vi "PUMP_feedback_P_FR.vi"(4 "Allow email":bool, 5 "FR Data":cluster{"time (s)":dbl, "volume (µl)":dbl}, 6 "t0":dbl, 7 "FRP":T1, 8 "error in":errorcluster, 9 "MFCS_EZ":T2, 10 "Volume setpoint":dbl, 11 "FR setpoint":dbl) -> (0 "error out":errorcluster, 1 "Allow email out":bool, 2 "FR Data OUT":cluster{"time (s)":dbl, "volume (µl)":dbl}, 3 "volume reached?":bool)   [LabVIEW 2015]
uses:
  <userlib>/Fluigent/Fluigent MFCS/FluigentMFCS_Full.llb/_EZmfcsRefNum.ctl
  <userlib>/Fluigent/Fluigent MFCS/FluigentMFCS_Full.llb/_EZmfcsEnum.ctl
  <userlib>/Fluigent/Fluigent FRP/FluigentFRP.llb/_frpEnum.ctl
  <userlib>/Fluigent/Fluigent MFCS/FluigentMFCS_Full.llb/MFCS_EZ Write Channel Pressure.vi
  GLOBAL/Global_MAIN.vi
panel:
  out "error out MAIL":errorcluster
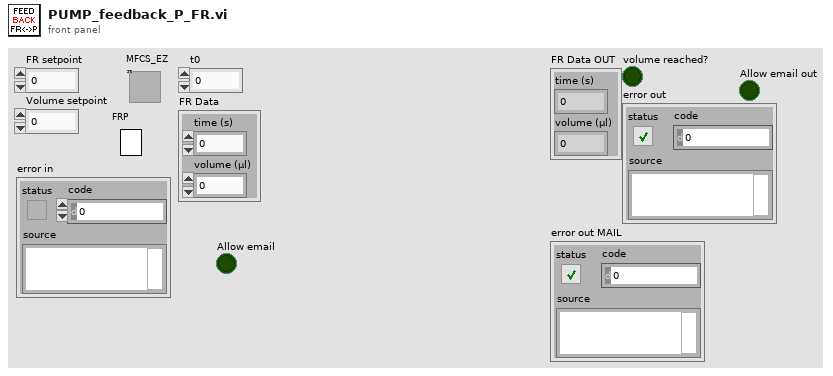
[diagram p1: front panel]
types:
  T1 = typedef "_frpRefNum" = refnum<k1>
  T2 = typedef "_EZmfcsRefNum.ctl" = refnum<k1>
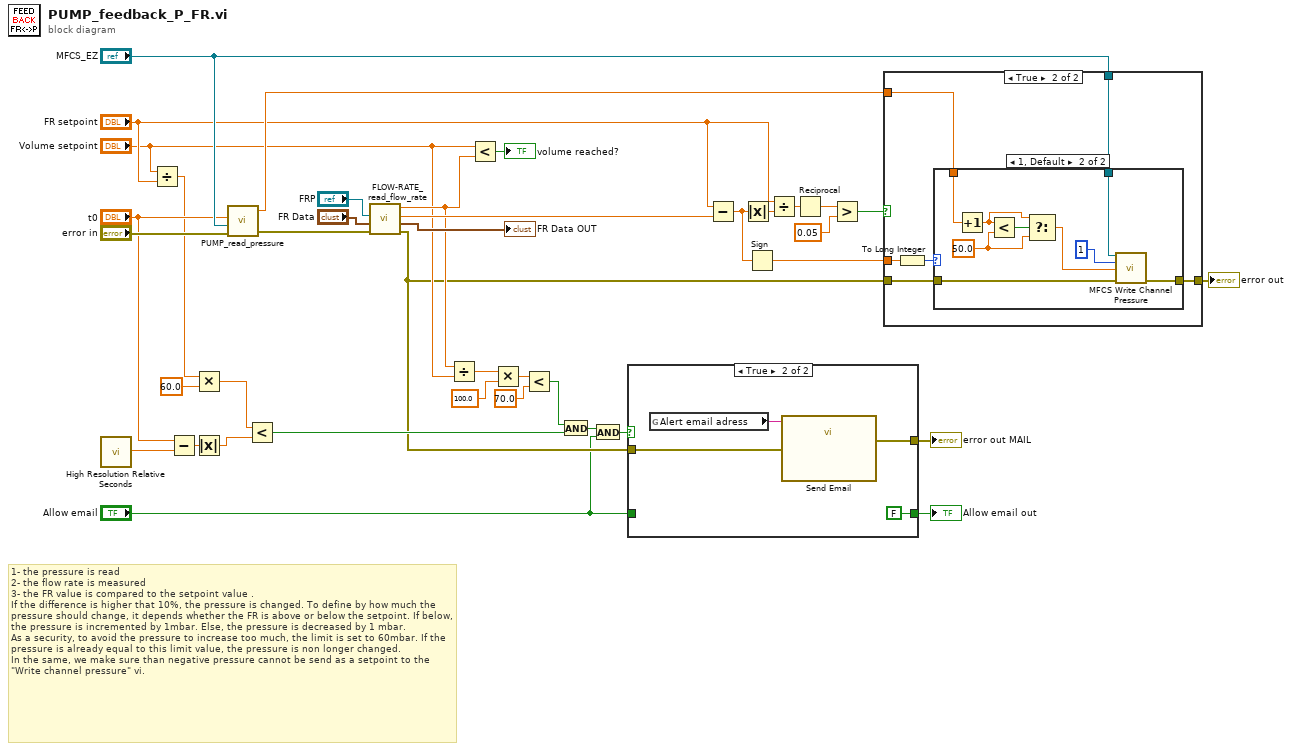
[diagram p0: block diagram]
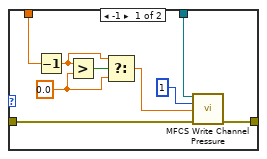
[diagram p4: hidden frame]
diagram:
  # "1- the pressure is read\n2- the flow rate is measured\n3- the FR value is compared to the setpoint value . \nIf the difference is higher that 10%, the pressure is changed. To define by how much the pressure should change, it depends whether the FR is above or below the setpoint. If below, the pressure is incremented by 1mbar. Else, the pressure is decreased by 1 mbar.\nAs a security, to avoid the pressure to increase too much, the limit is set to 60mbar. If the pressure is already equal to this limit value, the pressure is non longer changed.\nIn the same, we make sure than negative pressure cannot be send as a setpoint to the \"Write channel pressure\" vi."
  n1 = call <vilib>:"High Resolution Relative Seconds.vi"() -> ("relative seconds"=w21:dbl)
  n2 = Divide(x="Volume setpoint", y="FR setpoint") -> (x/y=w9:dbl)
  n3 = Subtract(x="t0", y=w21) -> (x-y=w19:dbl)
  n4 = Multiply(x=w9, y=60.0) -> (x*y=w7:dbl)
  n5 = Absolute Value(x=w19) -> (abs(x)=w18:dbl)
  n6 = call "PUMP_read_pressure.vi"("error in"="error in", "MFCS_EZ"="MFCS_EZ", "t0"="t0") -> ("error out"=w38:errorcluster, "Pressure (mBar)"=w27:dbl)  [unwired: 1 in, 1 out]
  n7 = Less?(x=w7, y=w18) -> (x < y?=w10:bool)
  n8 = call "FLOW-RATE_read_flow_rate.vi"("error in"=w38, "Data t i-1"="FR Data", "FRP out"="FRP") -> ("error out"=w6:errorcluster, "Data t i"=→"FR Data OUT":cluster{"time (s)":dbl, "volume (µl)":dbl}, "FR (µl/min)"=w35:dbl, "volume (µl)"=w17:dbl)  [unwired: 1 in]
  n9 = Divide(x=w17, y="Volume setpoint") -> (x/y=w15:dbl)
  n10 = Less?(x="Volume setpoint", y=w17) -> (x < y?=→"volume reached?":bool)
  n11 = Multiply(x=w15, y=100.0) -> (x*y=w13:dbl)
  n12 = Less?(x=w13, y=70.0) -> (x < y?=w11:bool)
  n13 = And(x=w11, y=w10) -> (x .and. y?=w4:bool)
  n14 = And(x=w4, y="Allow email") -> (x .and. y?=w3:bool)
  n15 = case shown="True" w3 {
    tunnel: w6 -> [w41 w44]
    tunnel: [w41 w43] -> w5
    tunnel: "Allow email" -> [w40 _]
    tunnel: [w40 FALSE ("Allow email")] -> w1
    frame False {
    }
    frame True {
      n16 = global read "Global_MAIN.vi" "Alert email adress"() -> (w45:string)
      n17 = call "Send Email"("error in"=w44, "Recipients"=w45) -> ("error out"=w43:errorcluster)  [unwired: 9 in]
    }
  }
  "error out MAIL" <- w5
  "Allow email out" <- w1
  n18 = Subtract(x="FR setpoint", y=w35) -> (x-y=w30:dbl)
  n19 = Absolute Value(x=w30) -> (abs(x)=w34:dbl)
  n20 = Sign(1:w30) -> (0:w29:dbl)
  n21 = Divide(x="FR setpoint", y=w34) -> (x/y=w33:dbl)
  n22 = Reciprocal(x=w33) -> (1/x=w32:dbl)
  n23 = Greater?(x=w32, y=0.05) -> (0:w26:bool)
  n24 = case shown="True" w26 {
    tunnel: w29 -> [_ w52]
    tunnel: w27 -> [_ w49]
    tunnel: "MFCS_EZ" -> [_ w50]
    tunnel: [w46 w48] -> w23
    tunnel: w6 -> [w46 w47]
    frame False {
    }
    frame True {
      n25 = To Long Integer(number=w52) -> (32bit integer=w51:i32)
      n26 = case shown="1, Default" w51 {
        tunnel: w50 -> [w61 w70]
        tunnel: w49 -> [w60 w69]
        tunnel: [w59 w68] -> w48
        tunnel: w47 -> [w53 w62]
        frame -1 {
          w56 = 0.0 ("y")
          n27 = Decrement(x=w60) -> (x-1=w57:dbl)
          n28 = Greater?(x=w57, y=w56) -> (0:w58:bool)
          n29 = Select(t=w57, s=w58, f=w56) -> (s? t:f=w55:dbl)
          n30 = call-poly <userlib>:"MFCS Write Channel Pressure.vi"("MFCS_EZ"=w61, "Channel Number (default=1)"=u8 1, "Pressure (mBar)"=w55, "error in (no error)"=w53) -> ("error out"=w59:errorcluster)  [unwired: 10 in, 1 out]
        }
        frame 1, Default {
          w65 = 50.0 ("y")
          n31 = Increment(x=w69) -> (x+1=w66:dbl)
          n32 = Less?(x=w66, y=w65) -> (x < y?=w67:bool)
          n33 = Select(t=w66, s=w67, f=w65) -> (s? t:f=w64:dbl)
          n34 = call-poly <userlib>:"MFCS Write Channel Pressure.vi"("MFCS_EZ"=w70, "Channel Number (default=1)"=u8 1, "Pressure (mBar)"=w64, "error in (no error)"=w62) -> ("error out"=w68:errorcluster)  [unwired: 10 in, 1 out]
        }
      }
    }
  }
  "error out" <- w23
